vi "RMS.vi"(10 "Number of samples":dbl, 11 "Array In":dbl[](array[numeric])) -> ()   [LabVIEW 2012]
panel:
  out "RMS":dbl
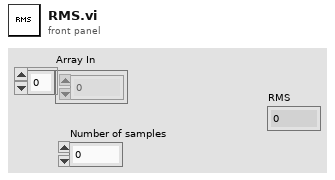
[diagram p1: front panel]
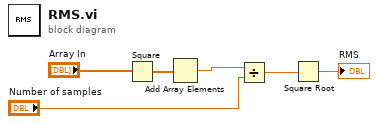
[diagram p0: block diagram]
diagram:
  n1 = Square(x="Array In") -> (x^2=w6:dbl[])
  n2 = Add Array Elements(numeric array=w6) -> (sum=w3:dbl)
  n3 = Divide(x=w3, y="Number of samples") -> (x/y=w5:dbl)
  n4 = Square Root(x=w5) -> (sqrt(x)=→"RMS":dbl)
